vi "Indent Subsquent Report.vi"(0 "report in":refnum<class "NI_HTML.lvclass">, 5 "level":i32, 11 "error in (no error)":errorcluster, 12 "MS Office parameters":T1) -> (4 "report out":refnum<class "NI_HTML.lvclass">, 15 "error out":errorcluster)   [LabVIEW 2017, in "NI_HTML.lvclass"]
uses:
  <vilib>/Utility/NIReport.llb/HTML/NI_HTML.lvclass
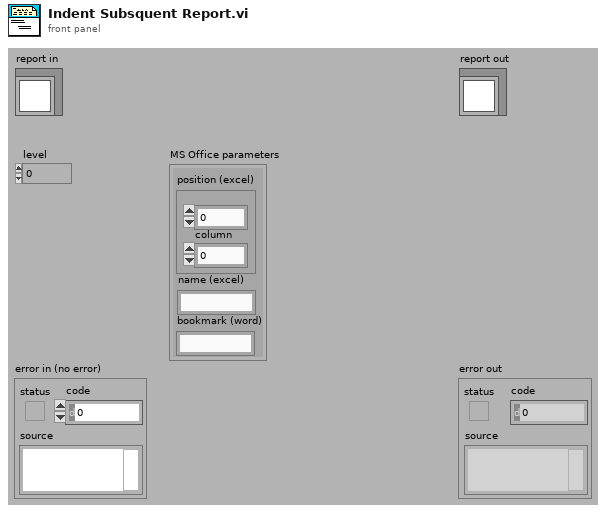
[diagram p1: front panel]
types:
  T1 = cluster{"position (excel)":cluster{"row":i32, "column":i32}, "name (excel)":string, "bookmark (word)":string}
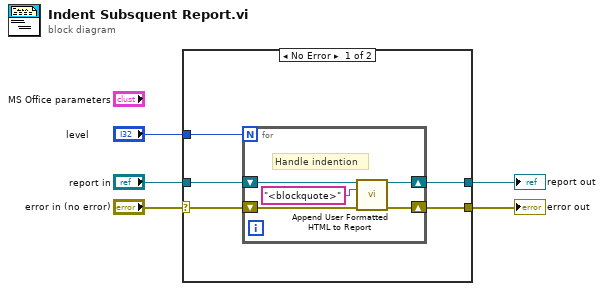
[diagram p0: block diagram]
diagram:
  n1 = case shown="No Error" "error in (no error)" {
    selector: "error in (no error)" -> [w7 w17]
    tunnel: [w6 w17] -> w4
    tunnel: [w9 w16] -> w2
    tunnel: "report in" -> [w10 w16]
    tunnel: "level" -> [w8 _]
    frame No Error {
      n2 = for {
        N: w8 -> [_]
        shift-right: [w12] -> w6
        shift-left: w7 -> [w13]
        shift-right: [w14] -> w9
        shift-left: w10 -> [w15]
        # "Handle indention"
        n3 = call-dynamic "Append User Formatted HTML to Report.vi"("report in"=w15, "HTML text"="<blockquote>" ("text"), "error in (no error)"=w13) -> ("report out"=w14:refnum<class "NI_HTML.lvclass">, "error out"=w12:errorcluster)  [unwired: 1 in, 10 out]
      }
    }
    frame Error {
    }
  }
  "error out" <- w4
  "report out" <- w2
